vi "Read Sinus penta5.vi"(9 "register values 2":u16[](array[numeric]), 10 "register values":u16[](array[numeric]), 11 "output cluster in":T1) -> (3 "output cluster out":T1)   [LabVIEW 2019]
uses:
  controls/Parametri inverter letti.ctl
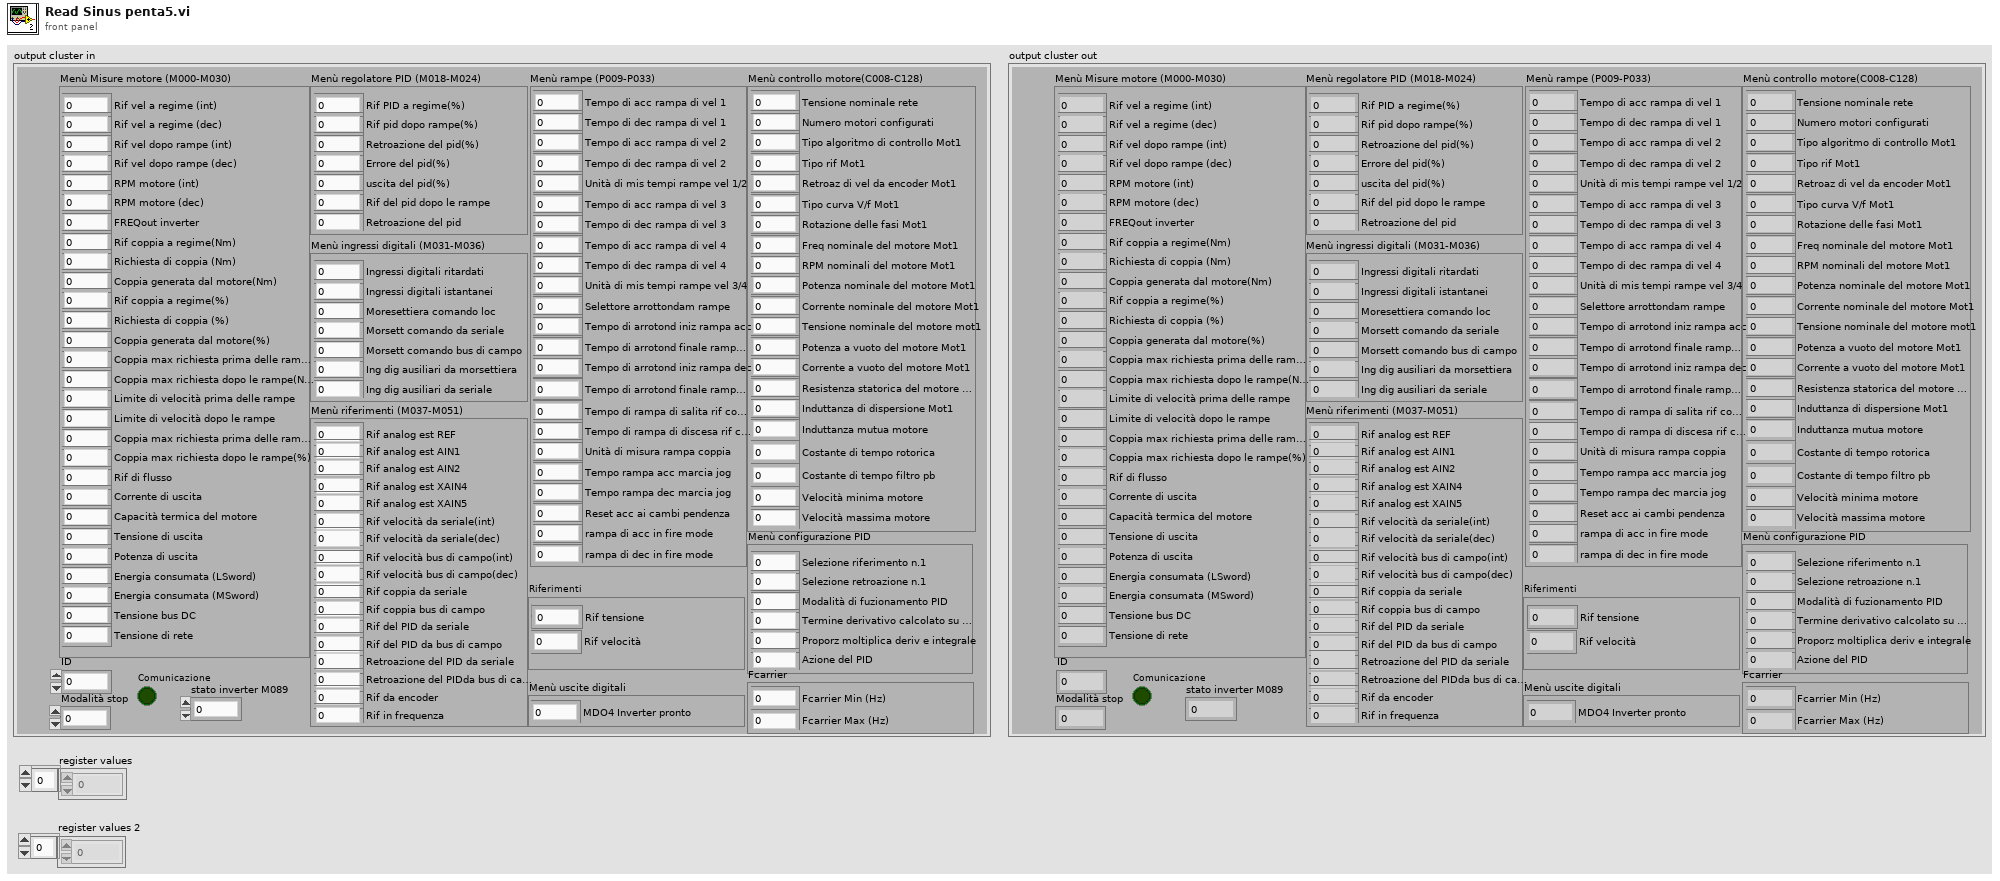
[diagram p1: front panel]
types:
  T1 = typedef "Parametri inverter letti.ctl" = cluster{"Menù Misure motore (M000-M030)":cluster{"Rif vel a regime (int)":u16, "Rif vel a regime (dec)":u16, "Rif vel dopo rampe (int)":u16, "Rif vel dopo rampe (dec)":u16, "RPM motore (int)":u16, "RPM motore (dec)":u16, "FREQout inverter":u16, "Rif coppia a regime(Nm)":u16, "Richiesta di coppia (Nm)":u16, "Coppia generata dal motore(Nm)":u16, "Rif coppia a regime(%)":u16, "Richiesta di coppia (%)":u16, "Coppia generata dal motore(%)":u16, "Coppia max richiesta prima delle rampe(Nm)":u16, "Coppia max richiesta dopo le rampe(Nm)":u16, "Limite di velocità prima delle rampe":u16, "Limite di velocità dopo le rampe":u16, "Coppia max richiesta prima delle rampe(%)":u16, "Coppia max richiesta dopo le rampe(%)":u16, "Rif di flusso":u16, "Corrente di uscita":u16, "Capacità termica del motore":u16, "Tensione di uscita":u16, "Potenza di uscita":u16, "Energia consumata (LSword)":u16, "Energia consumata (MSword)":u16, "Tensione bus DC":u16, "Tensione di rete":u16}, "Menù regolatore PID (M018-M024)":cluster{"Rif PID a regime(%)":u16, "Rif pid dopo rampe(%)":u16, "Retroazione del pid(%)":u16, "Errore del pid(%)":u16, "uscita del pid(%)":u16, "Rif del pid dopo le rampe":u16, "Retroazione del pid":u16}, "Menù ingressi digitali (M031-M036)":cluster{"Ingressi digitali ritardati":u16, "Ingressi digitali istantanei":u16, "Moresettiera comando loc":u16, "Morsett comando da seriale":u16, "Morsett comando bus di campo":u16, "Ing dig ausiliari da morsettiera":u16, "Ing dig ausiliari da seriale":u16}, "Menù riferimenti (M037-M051)":cluster{"Rif analog est REF":u16, "Rif analog est AIN1":u16, "Rif analog est AIN2":u16, "Rif analog est XAIN4":u16, "Rif analog est XAIN5":u16, "Rif velocità da seriale(int)":u16, "Rif velocità bus di campo(int)":u16, "Rif coppia da seriale":u16, "Rif coppia bus di campo":u16, "Rif del PID da seriale":u16, "Rif del PID da bus di campo":u16, "Retroazione del PID da seriale":u16, "Retroazione del PIDda bus di campo":u16, "Rif da encoder":u16, "Rif in frequenza":u16, "Rif velocità da seriale(dec)":u16, "Rif velocità bus di campo(dec)":u16}, "Menù rampe (P009-P033)":cluster{"Tempo di dec rampa di vel 1":u16, "Tempo di acc rampa di vel 2":u16, "Tempo di dec rampa di vel 2":u16, "Tempo di acc rampa di vel 1":u16, "Unità di mis tempi rampe vel 1/2":u16, "Tempo di acc rampa di vel 3":u16, "Tempo di dec rampa di vel 3":u16, "Tempo di acc rampa di vel 4":u16, "Tempo di dec rampa di vel 4":u16, "Unità di mis tempi rampe vel 3/4":u16, "Selettore arrottondam rampe":u16, "Tempo di arrotond iniz rampa acc":u16, "Tempo di arrotond finale rampa acc":u16, "Tempo di arrotond iniz rampa dec":u16, "Tempo di rampa di salita rif coppia":u16, "Tempo di rampa di discesa rif coppia":u16, "Unità di misura rampa coppia":u16, "Tempo rampa acc marcia jog":u16, "Tempo rampa dec marcia jog":u16, "Reset acc ai cambi pendenza":u16, "rampa di acc in fire mode":u16, "rampa di dec in fire mode":u16, "Tempo di arrotond finale rampa dec":u16}, "Menù controllo motore(C008-C128)":cluster{"Numero motori configurati":u16, "Tipo algoritmo di controllo Mot1":u16, "Tipo rif Mot1":u16, "Tensione nominale rete":u16, "Retroaz di vel da encoder Mot1":u16, "Tipo curva V/f Mot1":u16, "Rotazione delle fasi Mot1":u16, "Freq nominale del motore Mot1":u16, "RPM nominali del motore Mot1":u16, "Potenza nominale del motore Mot1":u16, "Corrente nominale del motore Mot1":u16, "Tensione nominale del motore mot1":u16, "Potenza a vuoto del motore Mot1":u16, "Corrente a vuoto del motore Mot1":u16, "Resistenza statorica del motore Mot1":u16, "Induttanza di dispersione Mot1":u16, "Induttanza mutua motore":u16, "Costante di tempo rotorica":u16, "Costante di tempo filtro pb":u16, "Velocità minima motore":u16, "Velocità massima motore":u16}, "Menù configurazione PID":cluster{"Selezione riferimento n.1":u16, "Selezione retroazione n.1":u16, "Modalità di fuzionamento PID":u16, "Termine derivativo calcolato su err o mis":u16, "Proporz moltiplica deriv e integrale":u16, "Azione del PID":u16}, "ID":dbl, "Menù uscite digitali":cluster{"MDO4 Inverter pronto":u16}, "Fcarrier":cluster{"Fcarrier Min (Hz)":u16, "Fcarrier Max (Hz)":u16}, "stato inverter M089":dbl, "Riferimenti":cluster{"Rif tensione":u16, "Rif velocità":u16}, "Comunicazione":bool, "Modalità stop":dbl}
  T2 = cluster{"Fcarrier Min (Hz)":u16, "Fcarrier Max (Hz)":u16}
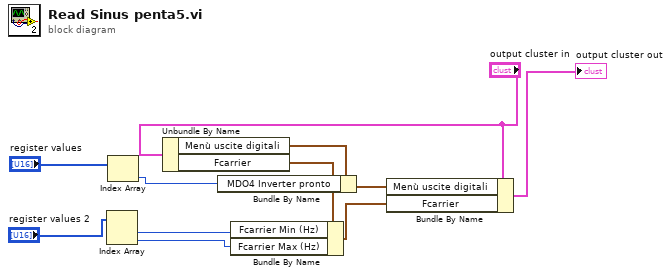
[diagram p0: block diagram]
diagram:
  n1 = Index Array(array="register values 2") -> (element #1=w2:u16, element #2=w1:u16)  [unwired: 2 in]
  n2 = Index Array(array="register values") -> (element=w8:u16)  [unwired: 1 in]
  n3 = Unbundle By Name("output cluster in") -> ("Menù uscite digitali"=w6:cluster{"MDO4 Inverter pronto":u16}, "Fcarrier"=w5:T2)
  n4 = Bundle By Name(cluster=w6, "MDO4 Inverter pronto"=w8) -> (w9:cluster{"MDO4 Inverter pronto":u16})
  n5 = Bundle By Name(cluster=w5, "Fcarrier Min (Hz)"=w2, "Fcarrier Max (Hz)"=w1) -> (w4:T2)
  n6 = Bundle By Name(cluster="output cluster in", "Menù uscite digitali"=w9, "Fcarrier"=w4) -> (→"output cluster out":T1)
